vi "Adam_server_messages.vi"(1 "Filename":path) -> ()   [LabVIEW 2021]
panel:
  out "String":string
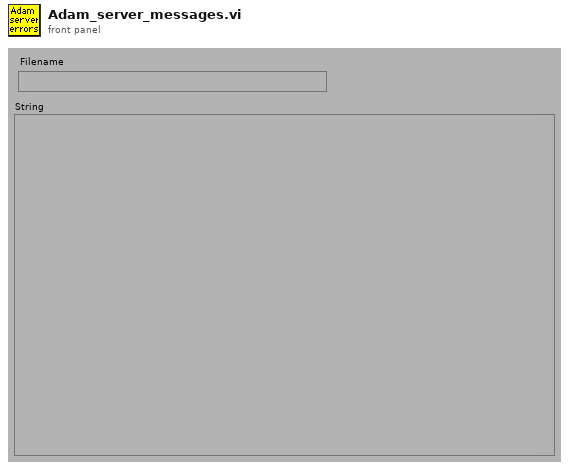
[diagram p1: front panel]
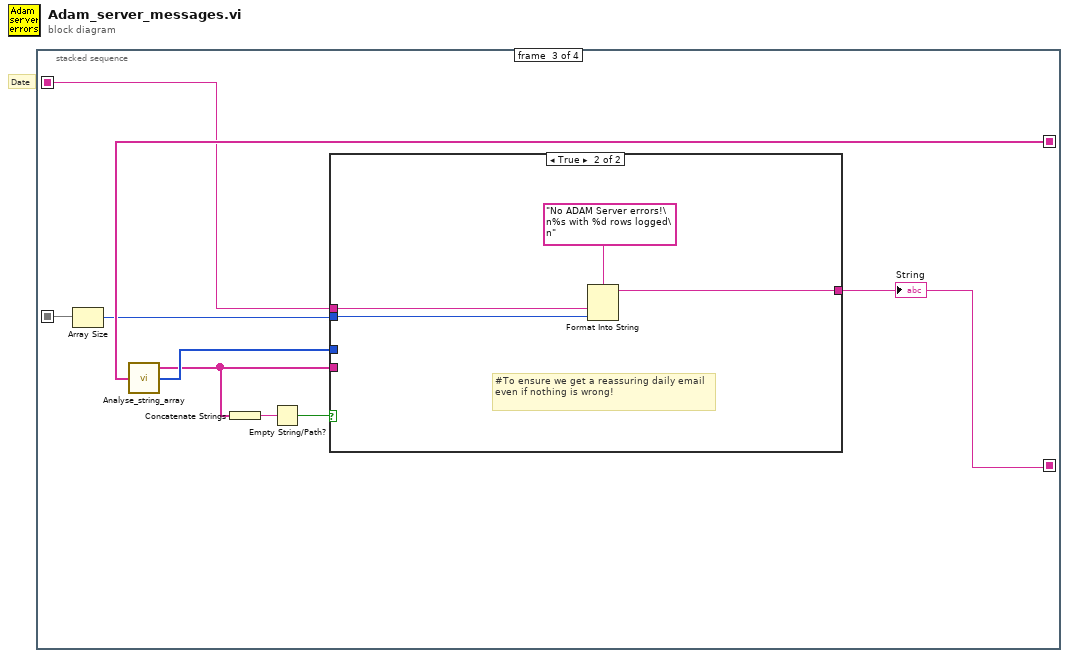
[diagram p0: block diagram]
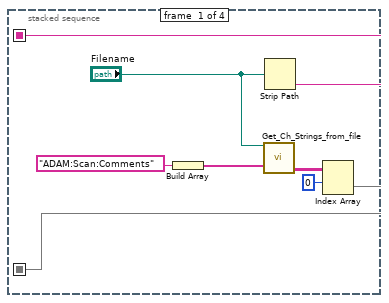
[diagram p2: hidden frame]
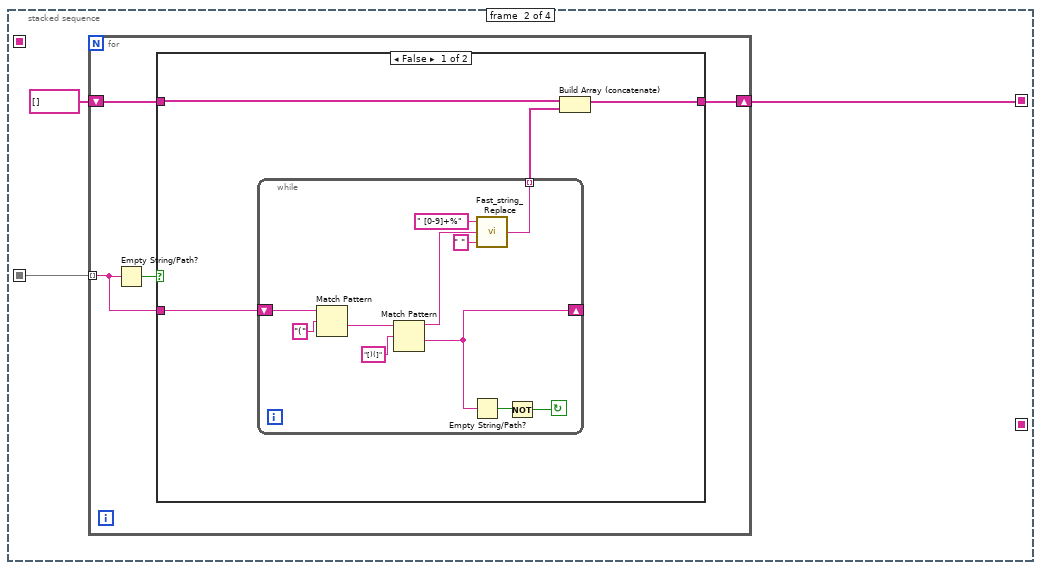
[diagram p3: hidden frame]
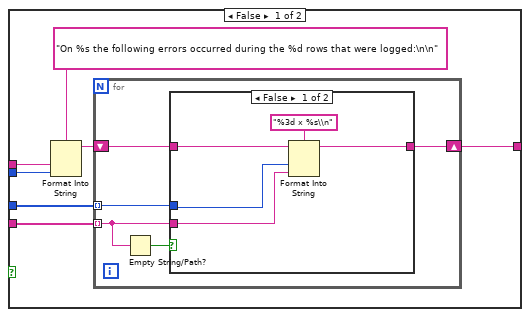
[diagram p5: hidden frame]
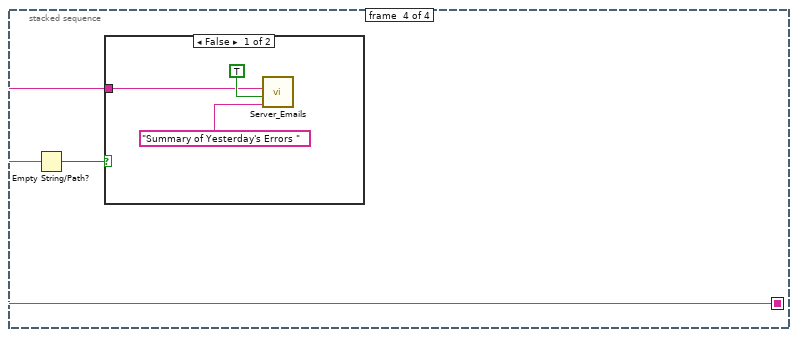
[diagram p7: hidden frame]
diagram:
  # "Date"
  n1 = stacked-sequence {
    seq-local: [w3 _ _ _] -> [_ w10 w37 _]
    seq-local: [_ w8 _ _] -> [_ _ w39 _]
    seq-local: [w2 _ _ _] -> [_ _ w33 _]
    seq-local: [_ _ w31 _] -> [_ _ _ w62]
    frame #0 {
      n2 = Build Array("ADAM:Scan:Comments") -> (w6:string[])
      n3 = call "Get_Ch_Strings_from_file.vi"("Filename"="Filename", "Channel names"=w6) -> ("Ch Data"=w4:string[][])  [unwired: 1 in, 12 out]
      n4 = Strip Path(path="Filename") -> (name=w2:string)  [unwired: 1 out]
      n5 = Index Array(array=w4, index (row)=0 ("Index")) -> (element=w3:string[])  [unwired: 1 in]
    }
    frame #1 {
      n6 = for {
        shift-right: [w13] -> w8
        shift-left: string[] [] -> [w12]
        tunnel: w10 -> [w11] mode=indexing
        n7 = Empty String/Path?(string/path=w11) -> (empty?=w14:bool)
        n8 = case shown="False" w14 {
          tunnel: [w15 w30] -> w13
          tunnel: w12 -> [w16 w30]
          tunnel: w11 -> [w18 _]
          frame False {
            n9 = while {
              tunnel: [w20] -> w17 mode=indexing
              shift-left: w18 -> [w28]
              shift-right: [w25] -> _
              stop <- w23 continue-if-true
              n10 = Match Pattern(string=w28, regular expression="(") -> (after substring=w26:string)  [unwired: 4 out]
              n11 = Match Pattern(string=w26, regular expression="[)(]") -> (before substring=w22:string, after substring=w25:string)  [unwired: 3 out]
              n12 = Empty String/Path?(string/path=w25) -> (empty?=w24:bool)
              n13 = call "Fast_string_Replace.vi"("Replace match with:"=" ", "Input String"=w22, "regular expression"=" [0-9]+%") -> ("Output String"=w20:string)  [unwired: 2 out]
              n14 = Not(x=w24) -> (.not. x?=w23:bool)
            }
            n15 = Build Array (concatenate)(w16, w17) -> (w15:string[])
          }
          frame True {
          }
        }
      }
    }
    frame #2 {
      n16 = Array Size(array=w37) -> (size(s)=w36:i32)
      n17 = call "Analyse_string_array.vi"("String array"=w39) -> ("Unique strings"=w35:string[], "Frequency"=w38:i32[])  [unwired: 1 out]
      n18 = Concatenate Strings(w35) -> (w34:string)
      n19 = Empty String/Path?(string/path=w34) -> (empty?=w32:bool)
      n20 = case shown="True" w32 {
        tunnel: w38 -> [w46 _]
        tunnel: w36 -> [w44 w60]
        tunnel: w35 -> [w42 _]
        tunnel: [w41 w58] -> w31
        tunnel: w33 -> [w40 w59]
        frame False {
          n21 = Format Into String(format string="On %s the following errors occurred during the %d rows that were logged:\n\n" ("Format String"), w40, w44) -> (resulting string=w43:string)  [unwired: 2 in, 1 out]
          n22 = for {
            tunnel: w42 -> [w48] mode=indexing
            tunnel: w46 -> [w51] mode=indexing
            shift-right: [w49] -> w41
            shift-left: w43 -> [w50]
            n23 = Empty String/Path?(string/path=w48) -> (empty?=w47:bool)
            n24 = case shown="False" w47 {
              tunnel: w51 -> [w52 _]
              tunnel: w50 -> [w56 w57]
              tunnel: [w55 w57] -> w49
              tunnel: w48 -> [w53 _]
              frame False {
                n25 = Format Into String(format string="%3d x %s\\n" ("Format String"), initial string=w56, w52, w53) -> (resulting string=w55:string)  [unwired: 1 in, 1 out]
              }
              frame True {
              }
            }
          }
        }
        frame True {
          # "#To ensure we get a reassuring daily email even if nothing is wrong!"
          n26 = Format Into String(format string="No ADAM Server errors!\n%s with %d rows logged\n" ("Format String"), w59, w60) -> (resulting string=w58:string)  [unwired: 2 in, 1 out]
        }
      }
      "String" <- w31
    }
    frame #3 {
      n27 = Empty String/Path?(string/path=w62) -> (empty?=w63:bool)
      n28 = case shown="False" w63 {
        tunnel: w62 -> [w64 _]
        frame False {
          n29 = call "Server_Emails.vi"("Message"=w64, "Contact All clients?"=TRUE, "Subject"="Summary of Yesterday's Errors ") -> ()  [unwired: 2 in, 3 out]
        }
        frame True {
        }
      }
    }
  }
